vi "限幅器（STR）.vi"(3 "下限":string, 4 "X_in":string, 5 "上限":string) -> (1 "X_Out":string)   [LabVIEW 2012]
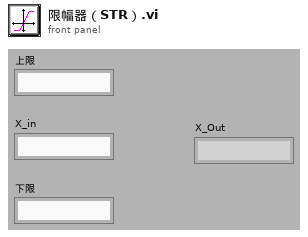
[diagram p1: front panel]
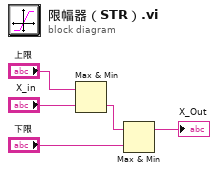
[diagram p0: block diagram]
diagram:
  n1 = Max & Min(x="上限", y="X_in") -> (min(x,y)=w3:string)  [unwired: 1 out]
  n2 = Max & Min(x=w3, y="下限") -> (max(x,y)=→"X_Out":string)  [unwired: 1 out]
